vi "FPGA_sbFOG.vi"() -> ()   [LabVIEW 2017]
uses:
  <vilib>/LabVIEW Targets/FPGA/cRIO/shared/nicrio_ModuleControls/nicrio_cRIO-9871_BaudRateEnum.ctl
  <vilib>/LabVIEW Targets/FPGA/cRIO/shared/nicrio_ModuleControls/nicrio_cRIO-9871_DataBitsEnum.ctl
  <vilib>/LabVIEW Targets/FPGA/cRIO/shared/nicrio_ModuleControls/nicrio_cRIO-9871_FlowControlEnum.ctl
  <vilib>/LabVIEW Targets/FPGA/cRIO/shared/nicrio_ModuleControls/nicrio_cRIO-9871_ParityEnum.ctl
  <vilib>/LabVIEW Targets/FPGA/cRIO/shared/nicrio_ModuleControls/nicrio_cRIO-9871_StopBitsEnum.ctl
  <vilib>/rvi/Emulation/niFpgaGetClockAttributes.vi
  <vilib>/rvi/Emulation/niFpgaSctlEmulationGetInTimedLoop.vi
  <vilib>/rvi/Emulation/niFpgaEmulationReportErrorSimple.vi
  <vilib>/rvi/eio/common/nirviEmuTemplatePropertySet_noerrors.vi
  <vilib>/rvi/eio/common/nirviEmuTemplateMethod_errors.vi
  <vilib>/rvi/Memory/Memory_Emulation/nirvimemoryEmulation.vi
  <vilib>/rvi/Memory/Memory_Emulation/nirvimemoryFastEmulation.vi
  <vilib>/rvi/DataTransferAndStorage/Container/Common/niFpgaContainerGetUniqueNameForEmu.vi
  <vilib>/rvi/Memory/Memory_Emulation/niFpgaMemoryEmulationCacheClearOnFirstRun.vi
  <vilib>/rvi/Memory/Memory_Emulation/nirvimemoryEmulationManagerCache_MakeExclusive.vi
  <vilib>/rvi/Memory/Memory_Emulation/niFpgaMemoryEmulationValidateCache.vi
  <vilib>/rvi/Memory/Memory_Emulation/nirvimemoryEmulationManagerCache_InsertValue.vi
  <vilib>/Utility/error.llb/Clear Errors.vi
  <vilib>/rvi/Memory/Memory_Emulation/nirvimemoryEmulationManagerCache_ReleaseExclusive.vi
  <vilib>/rvi/Memory/Memory_Emulation/nirvimemoryEmulationManagerCache_GetValue.vi
  <vilib>/rvi/Emulation/niFpgaEmulationIsFPGAContextNoSignature.vi
  <vilib>/rvi/Memory/Memory_Emulation/nirvimemoryEmulationManagerCache_SetValue.vi
  <vilib>/rvi/Emulation/niFpgaSctlEmulationResourceMgr.vi
  <vilib>/rvi/interface/RandomDataEmulation/niFpgaRandomDataHandleErrors.vi
  <vilib>/rvi/Emulation/niFpgaCriticalErrorInLSC.vi
  <vilib>/eio/EIOPropertyNode/EIOPropertyNode.xnode
  <vilib>/eio/EIOMethodNode/EIOMethodNode.xnode
  <vilib>/rvi/DataTransferAndStorage/Container/XNode/niFpgaContainer.xnode
  <vilib>/rvi/interface/RandomDataEmulation/nirviRandomDataFpgaReadWriteTemplate.vi
  <vilib>/eio/EIONode/EIONode.xnode
  <vilib>/rvi/eio/common/nirviEmuTemplatePropertyGet_errors.vi
  <vilib>/rvi/eio/common/nirviEmuTemplatePropertyGet_noerrors.vi
  <vilib>/rvi/eio/common/nirviEmuTemplatePropertySet_errors.vi
panel:
  in  "MIO/AO0":fxp<+/-,20,5>
  in  "MIO/AO1":fxp<+/-,20,5>
  in  "MIO/AO3":fxp<+/-,20,5>
  in  "MIO/AO2":fxp<+/-,20,5>
  out "MIO/DI_0":bool
  in  "MIO/DO_2":bool
  out "MIO/AI0..3":fxp<+/-,24,5>[](array[numeric])
  in  "MIO/DO_3":bool
  out "MIO/DI_1":bool
  in  "Count(uSec)":u32=1
  in  "Timeout_PW 4":i32=-1
  in  "Timeout_FW 4":i32=10
  out "CRC Check over Byte #10 to byte #29":bool
  out "CRC Check over Byte #2 to Byte #7":bool
  in  "Baud Rate_P2":T1=enum."115.2 kbps"
  in  "Timeout_PR 2":i32=-1
  in  "Timeout_FR 2":i32=10
  in  "Port2?":bool
  in  "Timeout_FW 3":i32=10
  in  "Timeout_PW 3":i32=-1
  in  "Bytes-to-Write P4":i32
  in  "Baud Rate_P4":T1=enum."115.2 kbps"
  in  "Op_Write P4":enum16{"Stand_by", "Write"}(ring)
  in  "Port4?":bool
  in  "Baud Rate_P1":T1=enum."115.2 kbps"
  in  "Timeout_PR 1":i32=-1
  in  "Timeout_FR 1":i32=10
  in  "Port1?":bool
  in  "Bytes-to-Write P3":i32
  in  "Baud Rate_P3":T1=enum."115.2 kbps"
  in  "Op_Write P3":enum16{"Stand_by", "Write"}(ring)
  in  "Port3?":bool
  # "TVA Read"
  # "DMARS Read"
  # "WRITE"
  # "WRITE"
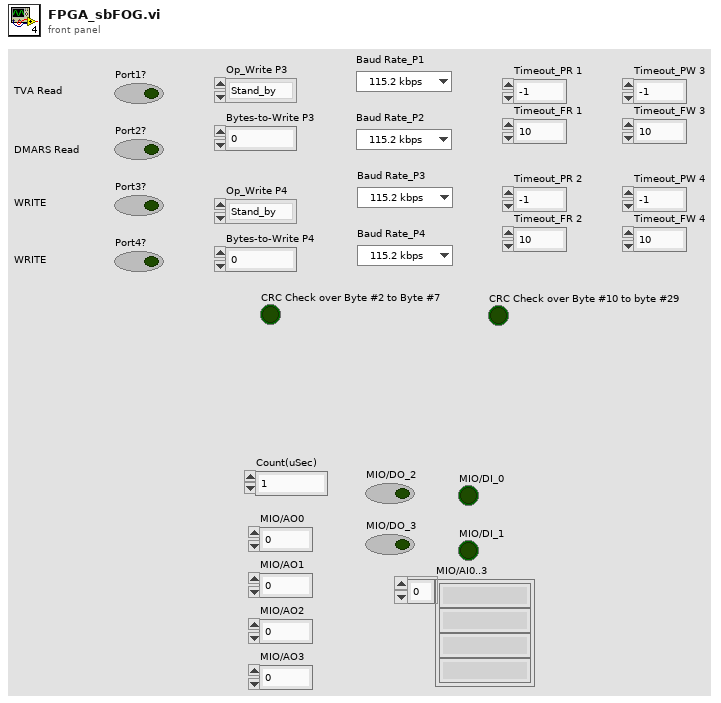
[diagram p1: front panel]
types:
  T1 = typedef "nicrio_cRIO-9871_BaudRateEnum.ctl" = enum16{"75 bps", "110 bps", "134 bps", "150 bps", "300 bps", "600 bps", "1200 bps", "1800 bps", "2400 bps", "4800 bps", "7200 bps", "9600 bps", "14.4 kbps", "19.2 kbps", "28.8 kbps", "38.4 kbps", "57.6 kbps", "115.2 kbps", "230.4 kbps", "460.8 kbps", "921.6 kbps"}
  T2 = typedef "nicrio_cRIO-9871_StopBitsEnum.ctl" = enum8{"1", "1.5", "2"}
  T3 = typedef "nicrio_cRIO-9871_ParityEnum.ctl" = enum8{"None", "Odd", "Even", "Mark", "Space"}
  T4 = typedef "nicrio_cRIO-9871_FlowControlEnum.ctl" = enum8{"None", "Software (XON / XOFF)", "Hardware (RTS / CTS)"}
  T5 = typedef "nicrio_cRIO-9871_DataBitsEnum.ctl" = enum8{"5", "6", "7", "8"}
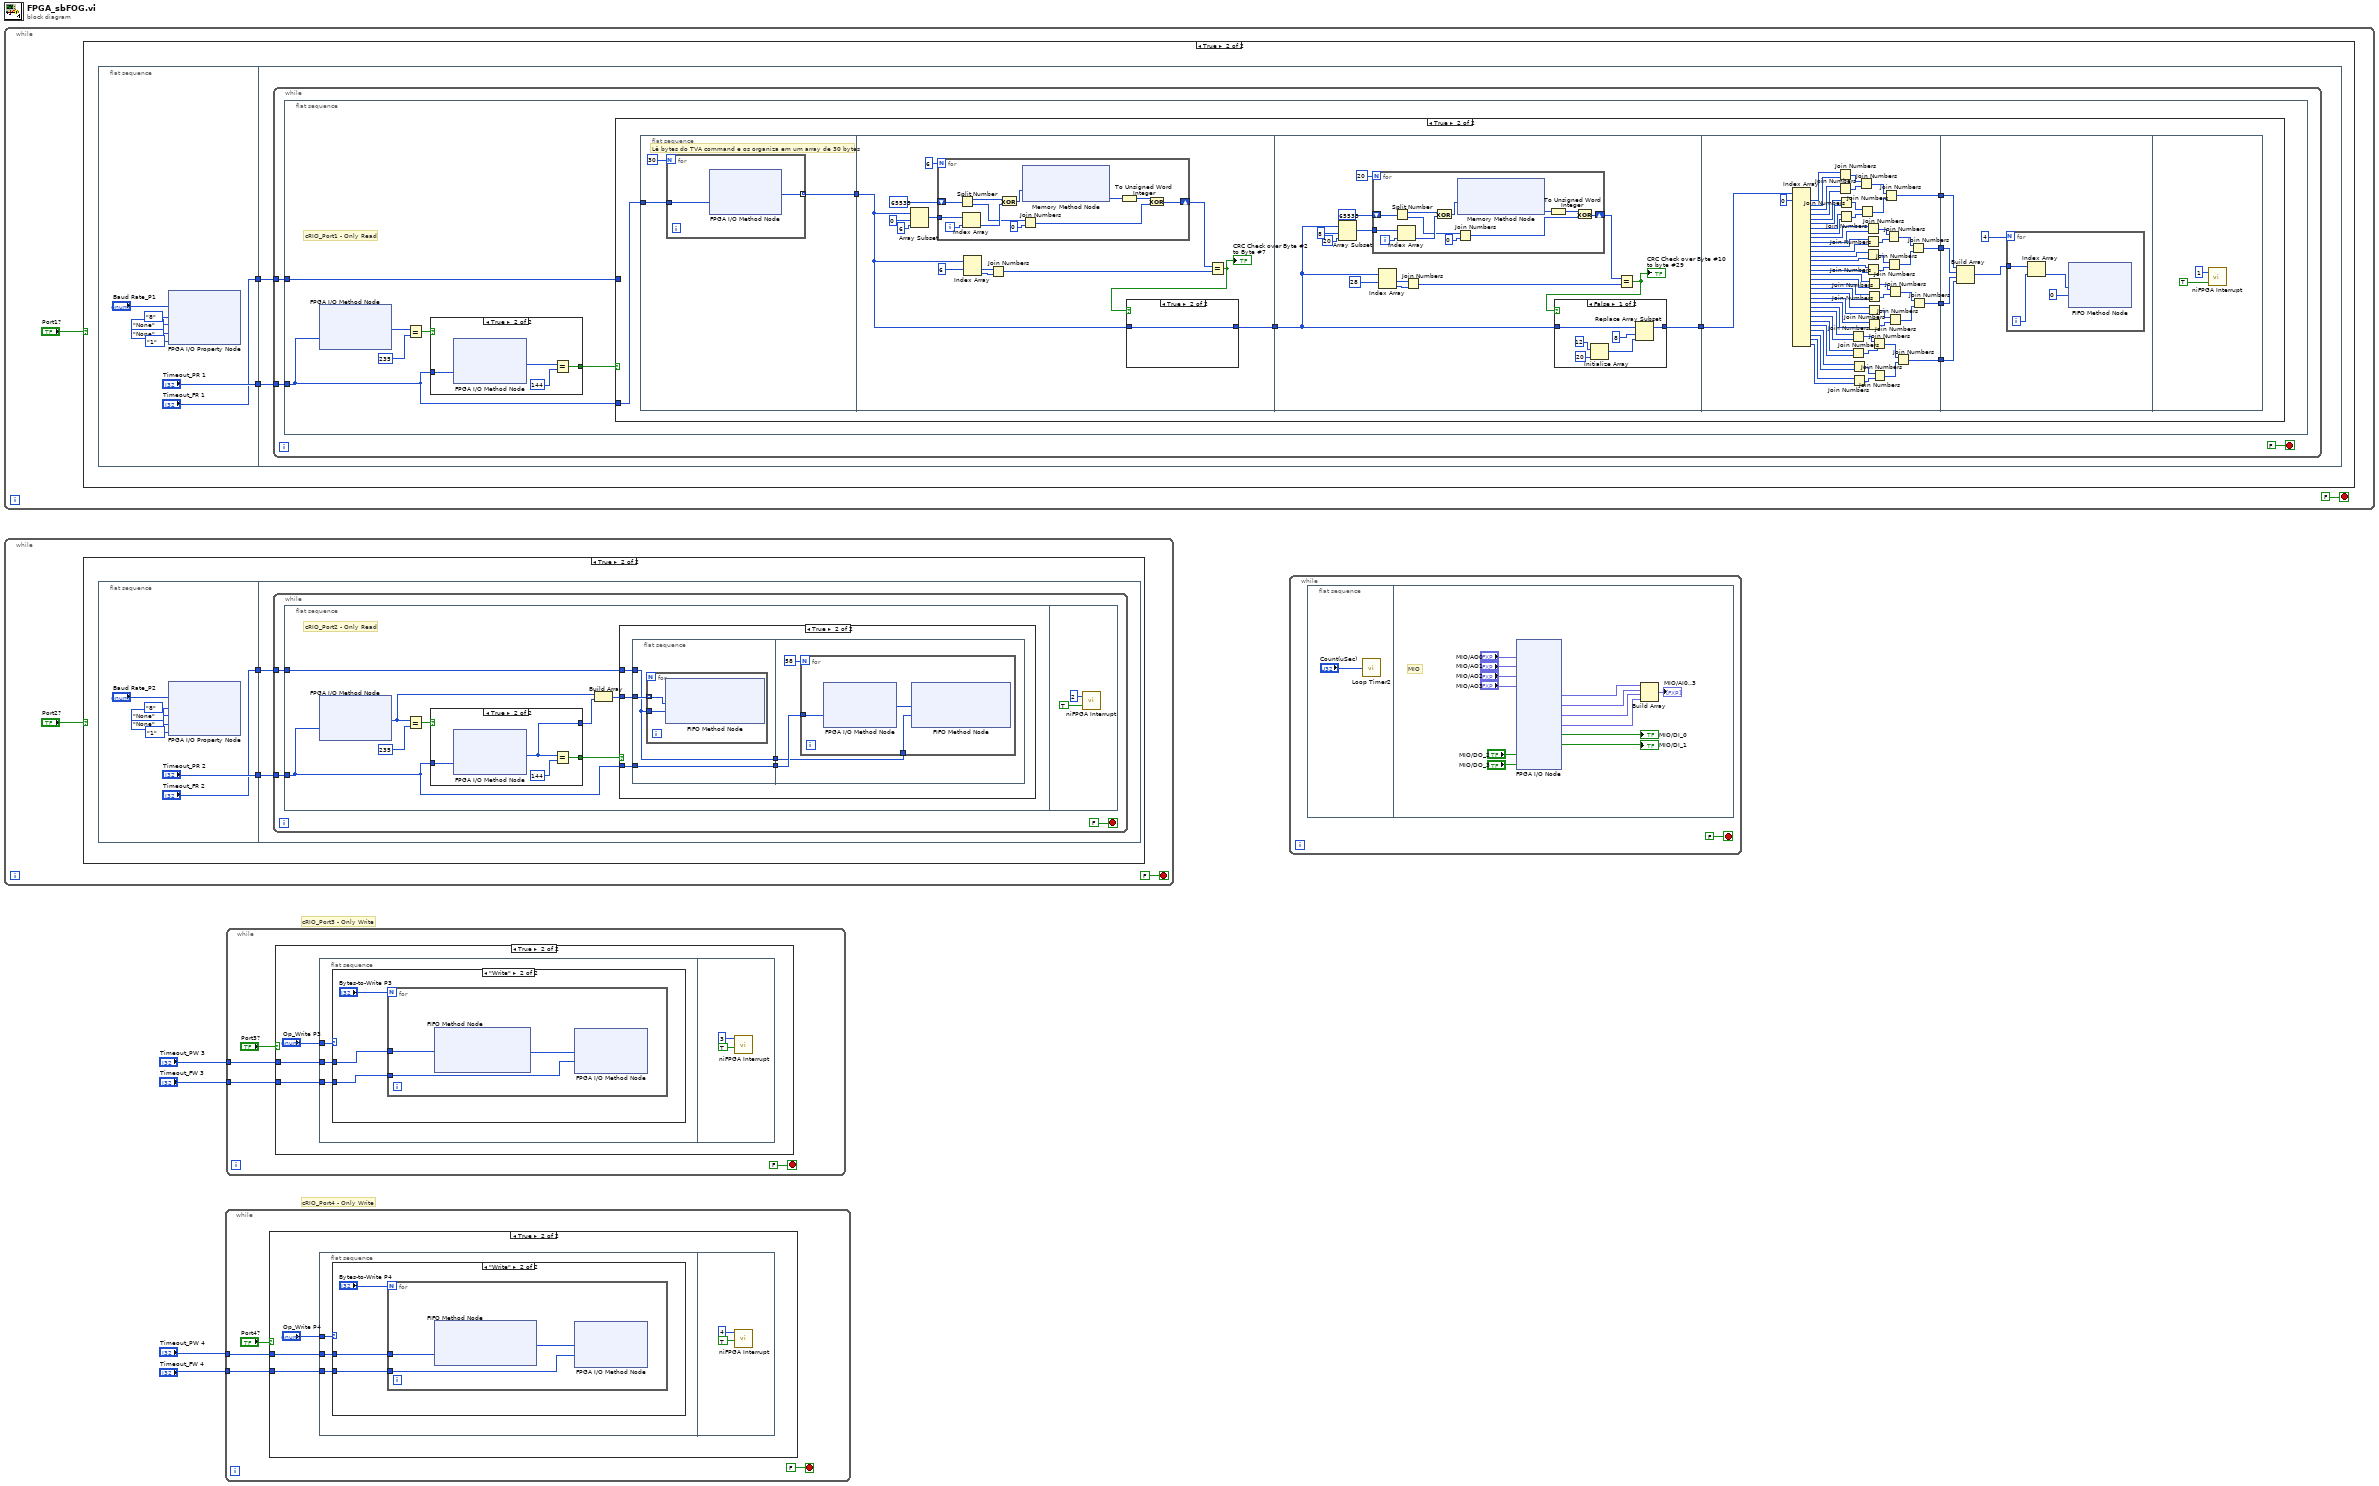
[diagram p0: block diagram]
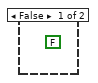
[diagram p3: hidden frame]
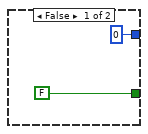
[diagram p4: hidden frame]
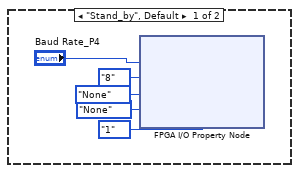
[diagram p6: hidden frame]
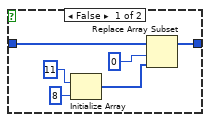
[diagram p9: hidden frame]
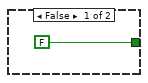
[diagram p11: hidden frame]
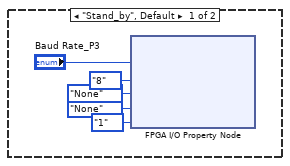
[diagram p13: hidden frame]
diagram:
  # "cRIO_Port4 - Only Write"
  # "cRIO_Port3 - Only Write"
  n1 = while {
    stop <- FALSE stop-if-true
    n2 = case shown="True" "Port1?" {
      frame False {
      }
      frame True {
        n3 = flat-sequence {
          tunnel: ["Timeout_PR 1"] -> w8
          tunnel: ["Timeout_FR 1"] -> w7
          tunnel: w8 -> [w17]
          tunnel: w7 -> [w16]
          frame #0 {
            n4 = xnode "FPGA I/O Property Node"("Baud Rate"="Baud Rate_P1", "Data Bits"=nicrio_cRIO-9871_DataBitsEnum."8", "Flow Control"=nicrio_cRIO-9871_FlowControlEnum."None", "Parity"=nicrio_cRIO-9871_ParityEnum."None", "Stop Bits"=nicrio_cRIO-9871_StopBitsEnum."1") -> ()  [unwired: 1 in, 1 out]
          }
          frame #1 {
            n5 = while {
              tunnel: w17 -> [w19]
              tunnel: w16 -> [w18]
              stop <- FALSE stop-if-true
              n6 = flat-sequence {
                tunnel: w19 -> [w23]
                tunnel: w18 -> [w22]
                frame #0 {
                  # "cRIO_Port1 - Only Read"
                  n7 = xnode "FPGA I/O Method Node"("Timeout (ms)"=w23) -> ("Data"=w24:u8)  [unwired: 1 in, 2 out]
                  n8 = Equal?(x=w24, y=u8 235) -> (x = y?=w25:bool)
                  n9 = case shown="True" w25 {
                    tunnel: [FALSE w181] -> w21
                    tunnel: w23 -> [_ w179]
                    frame False {
                    }
                    frame True {
                      n10 = xnode "FPGA I/O Method Node"("Timeout (ms)"=w179) -> ("Data"=w180:u8)  [unwired: 1 in, 2 out]
                      n11 = Equal?(x=w180, y=u8 144) -> (x = y?=w181:bool)
                    }
                  }
                  n12 = case shown="True" w21 {
                    tunnel: w23 -> [_ w27]
                    tunnel: w22 -> [_ _]
                    frame False {
                    }
                    frame True {
                      n13 = flat-sequence {
                        tunnel: [w36] -> w34
                        tunnel: w27 -> [w35]
                        tunnel: w34 -> [w42]
                        tunnel: [w41] -> w33
                        tunnel: [w73] -> w32
                        tunnel: w33 -> [w74]
                        tunnel: w32 -> [w108]
                        tunnel: [w107] -> w31
                        tunnel: [w106] -> w30
                        tunnel: [w105] -> w29
                        tunnel: [w104] -> w28
                        tunnel: w31 -> [w170]
                        tunnel: w30 -> [w169]
                        tunnel: w29 -> [w168]
                        tunnel: w28 -> [w167]
                        frame #0 {
                          # "Lê bytes do TVA command e os organiza em um array de 30 bytes"
                          n14 = for {
                            N: 30 -> [_]
                            tunnel: [w39] -> w36 mode=indexing
                            tunnel: w35 -> [w38]
                            n15 = xnode "FPGA I/O Method Node"("Timeout (ms)"=w38) -> ("Data"=w39:u8)  [unwired: 1 in, 2 out]
                          }
                        }
                        frame #1 {
                          n16 = Array Subset(array=w42, index=0, length=6) -> (w48:u8[])
                          n17 = for {
                            N: 6 -> [_]
                            tunnel: w48 -> [w71]
                            shift-right: [w63] -> w44
                            shift-left: u16 65535 ("index") -> [w67]
                            i -> [w70]
                            n18 = Split Number(x=w67) -> (hi(x)=w69:u8, lo(x)=w66:u8)
                            n19 = Index Array(array=w71, index=w70) -> (element=w68:u8)
                            n20 = Exclusive Or(1:w68, 2:w69) -> (0:w62:u8)
                            n21 = Join Numbers(hi=w66, lo=u8 0) -> ((hi.lo)=w64:u16)
                            n22 = xnode ("Memory Method Node")("Address"=w62) -> ("Data"=w61:i16)  [unwired: 1 in, 1 out]
                            n23 = To Unsigned Word Integer(number=w61) -> (unsigned 16bit integer=w60:u16)
                            n24 = Exclusive Or(1:w64, 2:w60) -> (0:w63:u16)
                          }
                          n25 = Index Array(array=w42, index #1=6 ("index")) -> (element #1=w46:u8, element #2=w45:u8)  [unwired: 1 in]
                          n26 = Join Numbers(hi=w46, lo=w45) -> ((hi.lo)=w43:u16)
                          n27 = Equal?(x=w44, y=w43) -> (x = y?=w40:bool)
                          "CRC Check over Byte #2 to Byte #7" <- w40
                          n28 = case shown="True" w40 {
                            tunnel: w42 -> [w54 w59]
                            tunnel: [w53 w59] -> w41
                            frame False {
                              n29 = Initialize Array(u8 11 ("element"), 8 ("dimension size")) -> (w55:u8[])
                              n30 = Replace Array Subset(array=w54, new element=w55, index=0) -> (w53:u8[])
                            }
                            frame True {
                            }
                          }
                        }
                        frame #2 {
                          n31 = Array Subset(array=w74, index=8, length=20) -> (w79:u8[])
                          n32 = for {
                            N: 20 -> [_]
                            tunnel: w79 -> [w103]
                            shift-right: [w95] -> w83
                            shift-left: u16 65535 ("index") -> [w99]
                            i -> [w102]
                            n33 = Split Number(x=w99) -> (hi(x)=w101:u8, lo(x)=w98:u8)
                            n34 = Index Array(array=w103, index=w102) -> (element=w100:u8)
                            n35 = Exclusive Or(1:w100, 2:w101) -> (0:w94:u8)
                            n36 = Join Numbers(hi=w98, lo=u8 0) -> ((hi.lo)=w96:u16)
                            n37 = xnode ("Memory Method Node")("Address"=w94) -> ("Data"=w93:i16)  [unwired: 1 in, 1 out]
                            n38 = To Unsigned Word Integer(number=w93) -> (unsigned 16bit integer=w92:u16)
                            n39 = Exclusive Or(1:w96, 2:w92) -> (0:w95:u16)
                          }
                          n40 = Index Array(array=w74, index #1=28 ("index")) -> (element #1=w81:u8, element #2=w82:u8)  [unwired: 1 in]
                          n41 = Join Numbers(hi=w81, lo=w82) -> ((hi.lo)=w84:u16)
                          n42 = Equal?(x=w83, y=w84) -> (x = y?=w72:bool)
                          "CRC Check over Byte #10 to byte #29" <- w72
                          n43 = case shown="False" w72 {
                            tunnel: w74 -> [w86 w91]
                            tunnel: [w85 w91] -> w73
                            frame False {
                              n44 = Initialize Array(u8 12 ("element"), 20 ("dimension size")) -> (w87:u8[])
                              n45 = Replace Array Subset(array=w86, new element=w87, index=8) -> (w85:u8[])
                            }
                            frame True {
                            }
                          }
                        }
                        frame #3 {
                          n46 = Index Array(array=w108, index #1=0 ("index")) -> (element #1=w110:u8, element #2=w111:u8, element #3=w112:u8, element #4=w113:u8, element #5=w118:u8, element #6=w119:u8, element #7=w120:u8, element #8=w121:u8, element #9=w130:u8, element #10=w131:u8, element #11=w132:u8, element #12=w133:u8, element #13=w134:u8, element #14=w135:u8, element #15=w136:u8, element #16=w137:u8, element #17=w144:u8, element #18=w145:u8, element #19=w146:u8, element #20=w147:u8, element #21=w148:u8, element #22=w149:u8, element #23=w150:u8, element #24=w151:u8, element #25=w158:u8, element #26=w159:u8, element #27=w160:u8, element #28=w161:u8, element #29=w162:u8, element #30=w163:u8, element #31=w164:u8, element #32=w165:u8)  [unwired: 31 in]
                          n47 = Join Numbers(hi=w110, lo=w111) -> ((hi.lo)=w114:u16)
                          n48 = Join Numbers(hi=w112, lo=w113) -> ((hi.lo)=w115:u16)
                          n49 = Join Numbers(hi=w118, lo=w119) -> ((hi.lo)=w117:u16)
                          n50 = Join Numbers(hi=w120, lo=w121) -> ((hi.lo)=w116:u16)
                          n51 = Join Numbers(hi=w158, lo=w159) -> ((hi.lo)=w152:u16)
                          n52 = Join Numbers(hi=w160, lo=w161) -> ((hi.lo)=w157:u16)
                          n53 = Join Numbers(hi=w162, lo=w163) -> ((hi.lo)=w155:u16)
                          n54 = Join Numbers(hi=w164, lo=w165) -> ((hi.lo)=w156:u16)
                          n55 = Join Numbers(hi=w114, lo=w115) -> ((hi.lo)=w122:u32)
                          n56 = Join Numbers(hi=w117, lo=w116) -> ((hi.lo)=w123:u32)
                          n57 = Join Numbers(hi=w130, lo=w131) -> ((hi.lo)=w129:u16)
                          n58 = Join Numbers(hi=w132, lo=w133) -> ((hi.lo)=w128:u16)
                          n59 = Join Numbers(hi=w134, lo=w135) -> ((hi.lo)=w126:u16)
                          n60 = Join Numbers(hi=w136, lo=w137) -> ((hi.lo)=w127:u16)
                          n61 = Join Numbers(hi=w144, lo=w145) -> ((hi.lo)=w143:u16)
                          n62 = Join Numbers(hi=w146, lo=w147) -> ((hi.lo)=w138:u16)
                          n63 = Join Numbers(hi=w148, lo=w149) -> ((hi.lo)=w140:u16)
                          n64 = Join Numbers(hi=w150, lo=w151) -> ((hi.lo)=w139:u16)
                          n65 = Join Numbers(hi=w152, lo=w157) -> ((hi.lo)=w154:u32)
                          n66 = Join Numbers(hi=w155, lo=w156) -> ((hi.lo)=w153:u32)
                          n67 = Join Numbers(hi=w122, lo=w123) -> ((hi.lo)=w107:u64)
                          n68 = Join Numbers(hi=w129, lo=w128) -> ((hi.lo)=w125:u32)
                          n69 = Join Numbers(hi=w126, lo=w127) -> ((hi.lo)=w124:u32)
                          n70 = Join Numbers(hi=w143, lo=w138) -> ((hi.lo)=w141:u32)
                          n71 = Join Numbers(hi=w140, lo=w139) -> ((hi.lo)=w142:u32)
                          n72 = Join Numbers(hi=w154, lo=w153) -> ((hi.lo)=w105:u64)
                          n73 = Join Numbers(hi=w125, lo=w124) -> ((hi.lo)=w106:u64)
                          n74 = Join Numbers(hi=w141, lo=w142) -> ((hi.lo)=w104:u64)
                        }
                        frame #4 {
                          n75 = Build Array(w170, w169, w167, w168) -> (w166:u64[])
                          n76 = for {
                            N: 4 -> [_]
                            tunnel: w166 -> [w174]
                            i -> [w175]
                            n77 = Index Array(array=w174, index=w175) -> (element=w172:u64)
                            n78 = xnode ("FIFO Method Node")("Element"=w172, "Timeout"=0) -> ()  [unwired: 1 in, 2 out]
                          }
                        }
                        frame #5 {
                          n79 = call <vilib>:"niFPGA Interrupt.vi"("Wait Until Cleared (F)"=TRUE, "IRQ Number (0)"=u8 1) -> ()  [unwired: 1 in]
                        }
                      }
                    }
                  }
                }
              }
            }
          }
        }
      }
    }
  }
  n80 = while {
    stop <- FALSE stop-if-true
    n81 = case shown="True" "Port2?" {
      frame False {
      }
      frame True {
        n82 = flat-sequence {
          tunnel: ["Timeout_PR 2"] -> w186
          tunnel: ["Timeout_FR 2"] -> w185
          tunnel: w186 -> [w195]
          tunnel: w185 -> [w194]
          frame #0 {
            n83 = xnode "FPGA I/O Property Node"("Baud Rate"="Baud Rate_P2", "Data Bits"=nicrio_cRIO-9871_DataBitsEnum."8", "Flow Control"=nicrio_cRIO-9871_FlowControlEnum."None", "Parity"=nicrio_cRIO-9871_ParityEnum."None", "Stop Bits"=nicrio_cRIO-9871_StopBitsEnum."1") -> ()  [unwired: 1 in, 1 out]
          }
          frame #1 {
            n84 = while {
              tunnel: w195 -> [w197]
              tunnel: w194 -> [w196]
              stop <- FALSE stop-if-true
              n85 = flat-sequence {
                tunnel: w197 -> [w200]
                tunnel: w196 -> [w199]
                frame #0 {
                  # "cRIO_Port2 - Only Read"
                  n86 = xnode "FPGA I/O Method Node"("Timeout (ms)"=w200) -> ("Data"=w201:u8)  [unwired: 1 in, 2 out]
                  n87 = Equal?(x=w201, y=u8 235) -> (x = y?=w203:bool)
                  n88 = case shown="True" w203 {
                    tunnel: [FALSE w227] -> w206
                    tunnel: [u8 0 ("Data") w226] -> w202
                    tunnel: w200 -> [_ w225]
                    frame False {
                    }
                    frame True {
                      n89 = xnode "FPGA I/O Method Node"("Timeout (ms)"=w225) -> ("Data"=w226:u8)  [unwired: 1 in, 2 out]
                      n90 = Equal?(x=w226, y=u8 144) -> (x = y?=w227:bool)
                    }
                  }
                  n91 = Build Array(w201, w202) -> (w205:u8[])
                  n92 = case shown="True" w206 {
                    tunnel: w205 -> [_ w211]
                    tunnel: w200 -> [_ w210]
                    tunnel: w199 -> [_ w207]
                    frame False {
                      (unwired) FALSE
                    }
                    frame True {
                      n93 = flat-sequence {
                        tunnel: w211 -> [w214]
                        tunnel: w210 -> [w213]
                        tunnel: [w213] -> w209
                        tunnel: [w212] -> w208
                        tunnel: w207 -> [w212]
                        tunnel: w209 -> [w218]
                        tunnel: w208 -> [w217]
                        frame #0 {
                          n94 = for {
                            tunnel: w214 -> [w216] mode=indexing
                            tunnel: w212 -> [w215]
                            n95 = xnode ("FIFO Method Node")("Element"=w216, "Timeout"=w215) -> ()  [unwired: 1 in, 2 out]
                          }
                        }
                        frame #1 {
                          n96 = for {
                            N: 58 -> [_]
                            tunnel: w218 -> [w221]
                            tunnel: w217 -> [w220]
                            n97 = xnode "FPGA I/O Method Node"("Timeout (ms)"=w221) -> ("Data"=w222:u8)  [unwired: 1 in, 2 out]
                            n98 = xnode ("FIFO Method Node")("Element"=w222, "Timeout"=w220) -> ()  [unwired: 1 in, 2 out]
                          }
                        }
                      }
                    }
                  }
                }
                frame #1 {
                  n99 = call <vilib>:"niFPGA Interrupt.vi"("Wait Until Cleared (F)"=TRUE, "IRQ Number (0)"=u8 2) -> ()  [unwired: 1 in]
                }
              }
            }
          }
        }
      }
    }
  }
  n100 = while {
    tunnel: "Timeout_PW 4" -> [w232]
    tunnel: "Timeout_FW 4" -> [w231]
    stop <- FALSE stop-if-true
    n101 = case shown="True" "Port4?" {
      tunnel: w232 -> [_ w236]
      tunnel: w231 -> [_ w235]
      frame False {
      }
      frame True {
        n102 = flat-sequence {
          tunnel: "Op_Write P4" -> [w240]
          tunnel: w236 -> [w239]
          tunnel: w235 -> [w238]
          frame #0 {
            n103 = case shown="\"Write\"" w240 {
              tunnel: w239 -> [_ w247]
              tunnel: w238 -> [_ w246]
              frame "Stand_by", Default {
                n104 = xnode "FPGA I/O Property Node"("Baud Rate"="Baud Rate_P4", "Data Bits"=nicrio_cRIO-9871_DataBitsEnum."8", "Flow Control"=nicrio_cRIO-9871_FlowControlEnum."None", "Parity"=nicrio_cRIO-9871_ParityEnum."None", "Stop Bits"=nicrio_cRIO-9871_StopBitsEnum."1") -> ()  [unwired: 1 in, 1 out]
              }
              frame "Write" {
                n105 = for {
                  N: "Bytes-to-Write P4" -> [_]
                  tunnel: w247 -> [w250]
                  tunnel: w246 -> [w249]
                  n106 = xnode ("FIFO Method Node")("Timeout"=w250) -> ("Element"=w251:u8)  [unwired: 1 in, 2 out]
                  n107 = xnode "FPGA I/O Method Node"("Data"=w251, "Timeout (ms)"=w249) -> ()  [unwired: 2 in, 3 out]
                }
              }
            }
          }
          frame #1 {
            n108 = call <vilib>:"niFPGA Interrupt.vi"("Wait Until Cleared (F)"=TRUE ("Wait Until Cleared"), "IRQ Number (0)"=u8 4 ("IRQ Number")) -> ()  [unwired: 1 in]
          }
        }
      }
    }
  }
  n109 = while {
    tunnel: "Timeout_PW 3" -> [w255]
    tunnel: "Timeout_FW 3" -> [w254]
    stop <- FALSE stop-if-true
    n110 = case shown="True" "Port3?" {
      tunnel: w255 -> [_ w259]
      tunnel: w254 -> [_ w258]
      frame False {
      }
      frame True {
        n111 = flat-sequence {
          tunnel: "Op_Write P3" -> [w263]
          tunnel: w259 -> [w262]
          tunnel: w258 -> [w261]
          frame #0 {
            n112 = case shown="\"Write\"" w263 {
              tunnel: w262 -> [_ w270]
              tunnel: w261 -> [_ w269]
              frame "Stand_by", Default {
                n113 = xnode "FPGA I/O Property Node"("Baud Rate"="Baud Rate_P3", "Data Bits"=nicrio_cRIO-9871_DataBitsEnum."8", "Flow Control"=nicrio_cRIO-9871_FlowControlEnum."None", "Parity"=nicrio_cRIO-9871_ParityEnum."None", "Stop Bits"=nicrio_cRIO-9871_StopBitsEnum."1") -> ()  [unwired: 1 in, 1 out]
              }
              frame "Write" {
                n114 = for {
                  N: "Bytes-to-Write P3" -> [_]
                  tunnel: w270 -> [w273]
                  tunnel: w269 -> [w272]
                  n115 = xnode ("FIFO Method Node")("Timeout"=w273) -> ("Element"=w274:u8)  [unwired: 1 in, 2 out]
                  n116 = xnode "FPGA I/O Method Node"("Data"=w274, "Timeout (ms)"=w272) -> ()  [unwired: 2 in, 3 out]
                }
              }
            }
          }
          frame #1 {
            n117 = call <vilib>:"niFPGA Interrupt.vi"("Wait Until Cleared (F)"=TRUE ("Wait Until Cleared"), "IRQ Number (0)"=u8 3 ("IRQ Number")) -> ()  [unwired: 1 in]
          }
        }
      }
    }
  }
  n118 = while {
    stop <- FALSE stop-if-true
    n119 = flat-sequence {
      frame #0 {
        n120 = call "Loop Timer2"("Count(uSec)"="Count(uSec)") -> ()  [unwired: 1 out]
      }
      frame #1 {
        # "MIO"
        n121 = xnode "FPGA I/O Node"("AO0"="MIO/AO0", "AO1"="MIO/AO1", "AO2"="MIO/AO2", "AO3"="MIO/AO3", "DIO2"="MIO/DO_2", "DIO3"="MIO/DO_3") -> ("AI0"=w291:fxp<+/-,24,5>, "AI1"=w290:fxp<+/-,24,5>, "AI2"=w289:fxp<+/-,24,5>, "AI3"=w288:fxp<+/-,24,5>, "DIO0"=→"MIO/DI_0":bool, "DIO1"=→"MIO/DI_1":bool)  [unwired: 12 in, 12 out]
        n122 = Build Array(w291, w290, w289, w288) -> (→"MIO/AI0..3":fxp<+/-,24,5>[])
      }
    }
  }
